vi "TxPkt - Init Packet Page.vi"(7 "Tx Packets Cluster In":T1, 8 "error in (no error)":errorcluster, 11 "Node Ptr In":T2 format="%.0x") -> (0 "error out":errorcluster, 3 "Node Ptr Out":T2 format="%.0x", 5 "Tx Packets Cluster Out":T1)   [LabVIEW 2019, in "UDP-Custom-Device System Explorer.lvlib"]
uses:
  UDP-Custom-Device System Explorer.lvlib
  <vilib>/NI VeriStand/Custom Device API/Custom Device Item Ref.ctl
  Types/Page References/Refs - Tx Packets Page.ctl
  <vilib>/NI VeriStand/Custom Device API/Custom Device API.lvlib
  Property Accessors/Tx Packet Accessors.lvlib
  Property Accessors/Shared Packet Accessors.lvlib
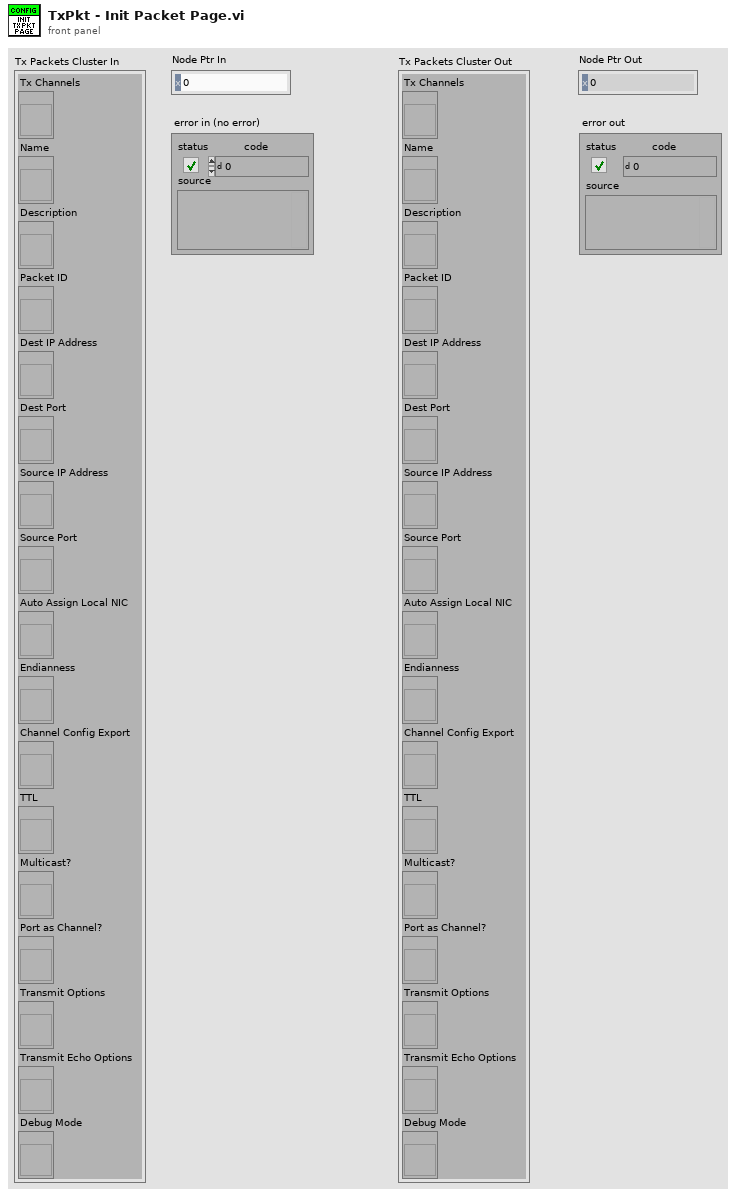
[diagram p1: front panel]
types:
  T1 = typedef "UDP-Custom-Device System Explorer.lvlib/Refs - Tx Packets Page.ctl" = cluster{"Tx Channels":refnum<vi>, "Name":refnum<vi>, "Description":refnum<vi>, "Packet ID":refnum<vi>, "Dest IP Address":refnum<vi>, "Dest Port":refnum<vi>, "Source IP Address":refnum<vi>, "Source Port":refnum<vi>, "Auto Assign Local NIC":refnum<vi>, "Endianness":refnum<vi>, "Channel Config Export":refnum<vi>, "TTL":refnum<vi>, "Multicast?":refnum<vi>, "Port as Channel?":refnum<vi>, "Transmit Options":refnum<vi>, "Transmit Echo Options":refnum<vi>, "Debug Mode":refnum<vi>}
  T2 = typedef "Custom Device API.lvlib/Custom Device Item Ref.ctl" = u64
  T3 = enum8{"Enabled", "Disabled", "Disabled and Grayed Out"}
  T4 = typedef "UDP-Custom-Device Shared.lvlib/Shared - Transmit Echo Options.ctl" = enum16{"PCL Reset", "Counter", "Mirror"}
  T5 = typedef "UDP-Custom-Device Shared.lvlib/Shared - Transmit Flag Options.ctl" = enum16{"Always", "One-Shot", "Toggle"}
  T6 = typedef "Custom Device API.lvlib/Custom Device Item Info.ctl" = cluster{"Name":string, "Is Channel":bool, "GUID":string, "Is Waveform":bool}
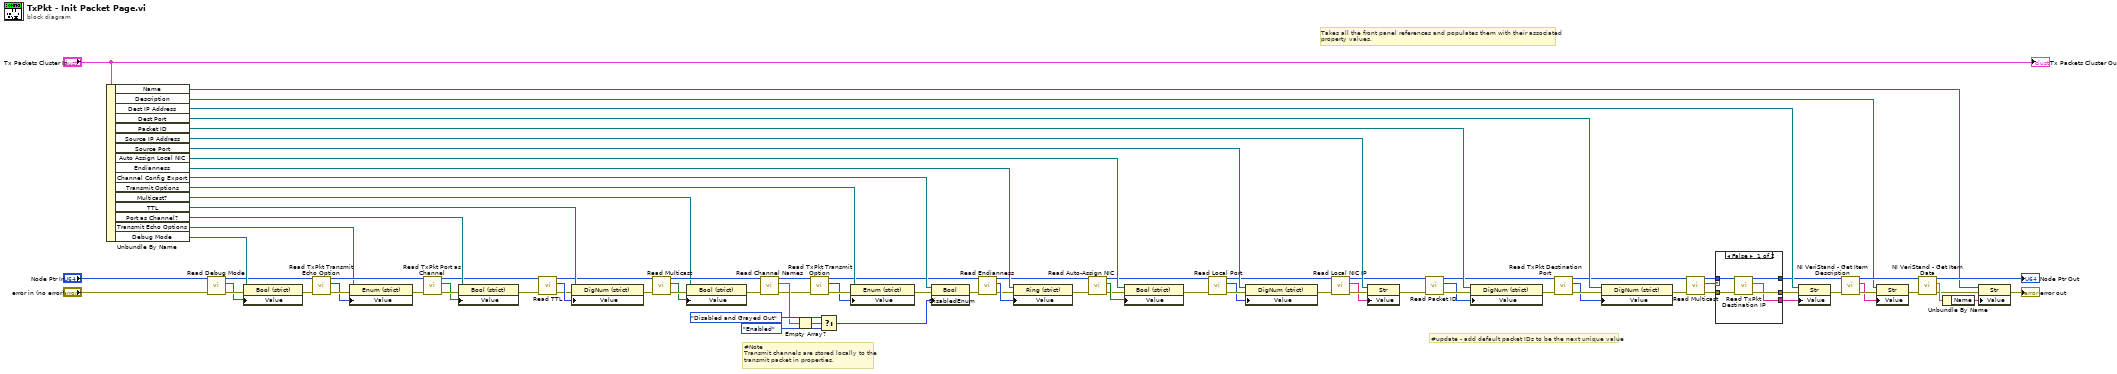
[diagram p0: block diagram]
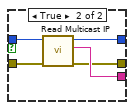
[diagram p2: hidden frame]
diagram:
  # "#Note\nTransmit channels are stored locally to the\ntransmit packet in properties."
  # "Takes all the front panel references and populates them with their associated\nproperty values."
  # "#update - add default packet IDs to be the next unique value"
  n1 = Unbundle By Name("Tx Packets Cluster In") -> ("Name"=w77:refnum<vi>, "Description"=w78:refnum<vi>, "Dest IP Address"=w80:refnum<vi>, "Dest Port"=w81:refnum<vi>, "Packet ID"=w82:refnum<vi>, "Source IP Address"=w76:refnum<vi>, "Source Port"=w75:refnum<vi>, "Auto Assign Local NIC"=w74:refnum<vi>, "Endianness"=w53:refnum<vi>, "Channel Config Export"=w48:refnum<vi>, "Transmit Options"=w41:refnum<vi>, "Multicast?"=w33:refnum<vi>, "TTL"=w39:refnum<vi>, "Port as Channel?"=w23:refnum<vi>, "Transmit Echo Options"=w13:refnum<vi>, "Debug Mode"=w9:refnum<vi>)
  n2 = call "Read Debug Mode.vi"("error in (no error)"="error in (no error)", "Node Ptr"="Node Ptr In") -> ("error out"=w4:errorcluster, "Debug Mode"=w3:bool, "Node Ptr out"=w6:T2)  [unwired: 7 in]
  n3 = property class="Bool (strict)"(reference=w9, error in=w4, "Value"=w3) -> (error out=w8:errorcluster)  [unwired: 1 out]
  n4 = call "Read TxPkt Transmit Echo Option.vi"("error in (no error)"=w8, "Node Ptr"=w6) -> ("error out"=w12:errorcluster, "Transmit Echo Options"=w10:T4, "Node Ptr out"=w14:T2)  [unwired: 7 in]
  n5 = property class="Enum (strict)"(reference=w13, error in=w12, "Value"=w10) -> (error out=w11:errorcluster)  [unwired: 1 out]
  n6 = call "Read TxPkt Port as Channel.vi"("error in (no error)"=w11, "Node Ptr"=w14) -> ("error out"=w21:errorcluster, "Port as Channel"=w20:bool, "Node Ptr out"=w22:T2)  [unwired: 7 in]
  n7 = property class="Bool (strict)"(reference=w23, error in=w21, "Value"=w20) -> (error out=w24:errorcluster)  [unwired: 1 out]
  n8 = call "Read TTL.vi"("error in (no error)"=w24, "Node Ptr"=w22) -> ("error out"=w37:errorcluster, "TTL"=w38:u16, "Node Ptr out"=w36:T2)  [unwired: 7 in]
  n9 = property class="DigNum (strict)"(reference=w39, error in=w37, "Value"=w38) -> (error out=w34:errorcluster)  [unwired: 1 out]
  n10 = call "Read Multicast.vi"("error in (no error)"=w34, "Node Ptr"=w36) -> ("error out"=w32:errorcluster, "Multicast"=w30:bool, "Node Ptr out"=w35:T2)  [unwired: 7 in]
  n11 = property class="Bool (strict)"(reference=w33, error in=w32, "Value"=w30) -> (error out=w31:errorcluster)  [unwired: 1 out]
  n12 = call "Read Channel Names.vi"("error in (no error)"=w31, "Node Ptr"=w35) -> ("error out"=w16:errorcluster, "Channel Names"=w43:string[], "Node Ptr out"=w19:T2)  [unwired: 7 in]
  n13 = Empty Array?(array=w43) -> (empty?=w44:bool)
  n14 = call "Read TxPkt Transmit Option.vi"("error in (no error)"=w16, "Node Ptr"=w19) -> ("error out"=w17:errorcluster, "Transmit Options"=w15:T5, "Node Ptr out"=w18:T2)  [unwired: 7 in]
  n15 = Select(t=T3."Disabled and Grayed Out" ("Disabled"), s=w44, f=T3."Enabled" ("Disabled")) -> (s? t:f=w42:T3)
  n16 = property class="Enum (strict)"(reference=w41, error in=w17, "Value"=w15) -> (error out=w40:errorcluster)  [unwired: 1 out]
  n17 = property class="Bool"(reference=w48, error in=w40, "DisabledEnum"=w42) -> (error out=w47:errorcluster)  [unwired: 1 out]
  n18 = call "Read Endianness.vi"("error in (no error)"=w47, "Node Ptr"=w18) -> ("error out"=w50:errorcluster, "Endianness"=w52:u16, "Node Ptr out"=w51:T2)  [unwired: 7 in]
  n19 = property class="Ring (strict)"(reference=w53, error in=w50, "Value"=w52) -> (error out=w49:errorcluster)  [unwired: 1 out]
  n20 = call "Read Auto-Assign NIC.vi"("error in (no error)"=w49, "Node Ptr"=w51) -> ("error out"=w71:errorcluster, "Auto-Assign NIC"=w72:bool, "Node Ptr out"=w70:T2)  [unwired: 7 in]
  n21 = property class="Bool (strict)"(reference=w74, error in=w71, "Value"=w72) -> (error out=w69:errorcluster)  [unwired: 1 out]
  n22 = call "Read Local Port.vi"("error in (no error)"=w69, "Node Ptr"=w70) -> ("error out"=w68:errorcluster, "Port"=w67:u16, "Node Ptr out"=w66:T2)  [unwired: 7 in]
  n23 = property class="DigNum (strict)"(reference=w75, error in=w68, "Value"=w67) -> (error out=w65:errorcluster)  [unwired: 1 out]
  n24 = call "Read Local NIC IP.vi"("error in (no error)"=w65, "Node Ptr"=w66) -> ("error out"=w64:errorcluster, "IP Address of Local NIC"=w63:string, "Node Ptr out"=w1:T2)  [unwired: 7 in]
  n25 = property class="Str"(reference=w76, error in=w64, "Value"=w63) -> (error out=w2:errorcluster)  [unwired: 1 out]
  n26 = call "Read Packet ID.vi"("error in (no error)"=w2, "Node Ptr"=w1) -> ("error out"=w62:errorcluster, "Packet ID"=w61:i32, "Node Ptr out"=w60:T2)  [unwired: 7 in]
  n27 = property class="DigNum (strict)"(reference=w82, error in=w62, "Value"=w61) -> (error out=w59:errorcluster)  [unwired: 1 out]
  n28 = call "Read TxPkt Destination Port.vi"("error in (no error)"=w59, "Node Ptr"=w60) -> ("error out"=w58:errorcluster, "Destination Port"=w57:u16, "Node Ptr out"=w27:T2)  [unwired: 7 in]
  n29 = property class="DigNum (strict)"(reference=w81, error in=w58, "Value"=w57) -> (error out=w29:errorcluster)  [unwired: 1 out]
  n30 = call "Read Multicast.vi"("error in (no error)"=w29, "Node Ptr"=w27) -> ("error out"=w28:errorcluster, "Multicast"=w25:bool, "Node Ptr out"=w26:T2)  [unwired: 7 in]
  n31 = case shown="False" w25 {
    tunnel: [w96 w99] -> w56
    tunnel: [w95 w97] -> w55
    tunnel: [w94 w98] -> w54
    tunnel: w28 -> [w93 w100]
    tunnel: w26 -> [w92 w101]
    frame False {
      n32 = call "Read TxPkt Destination IP.vi"("error in (no error)"=w93, "Node Ptr"=w92) -> ("error out"=w95:errorcluster, "Destination IP"=w94:string, "Node Ptr out"=w96:T2)  [unwired: 7 in]
    }
    frame True {
      n33 = call "Read Multicast IP.vi"("error in (no error)"=w100, "Node Ptr"=w101) -> ("error out"=w97:errorcluster, "Multicast IP Address"=w98:string, "Node Ptr out"=w99:T2)  [unwired: 7 in]
    }
  }
  n34 = property class="Str"(reference=w80, error in=w55, "Value"=w54) -> (error out=w73:errorcluster)  [unwired: 1 out]
  n35 = call <vilib>:"NI VeriStand - Get Item Description.vi"("error in (no error)"=w73, "Item Ref in"=w56) -> ("error out"=w89:errorcluster, "Description"=w88:string, "Item Ref out"=w86:T2)  [unwired: 7 out]
  n36 = property class="Str"(reference=w78, error in=w89, "Value"=w88) -> (error out=w87:errorcluster)  [unwired: 1 out]
  n37 = call <vilib>:"NI VeriStand - Get Item Data.vi"("error in (no error)"=w87, "Item Ref in"=w86) -> ("error out"=w90:errorcluster, "Item Info"=w91:T6, "Item Ref out"=→"Node Ptr Out":T2)  [unwired: 6 in, 1 out]
  n38 = Unbundle By Name(w91) -> ("Name"=w85:string)
  n39 = property class="Str"(reference=w77, error in=w90, "Value"=w85) -> (error out=→"error out":errorcluster)  [unwired: 1 out]
  "Tx Packets Cluster Out" <- "Tx Packets Cluster In"
